vi "Equipment.vi"(8 "Error In":errorcluster, 11 "Equipment in":T1) -> (0 "Error Out":errorcluster, 3 "Equipment out":T1)   [LabVIEW 2018]
uses:
  Equipment.ctl
panel:
  in  "IMEI":string caption="String"
  in  "Serial Number":string caption="String"
  in  "Manufacturer":string caption="String"
  in  "Model":string caption="String"
  in  "Trademark":string caption="String"
  in  "Equipment":string caption="String"
  in  "Save":bool
  # "Equipment:"
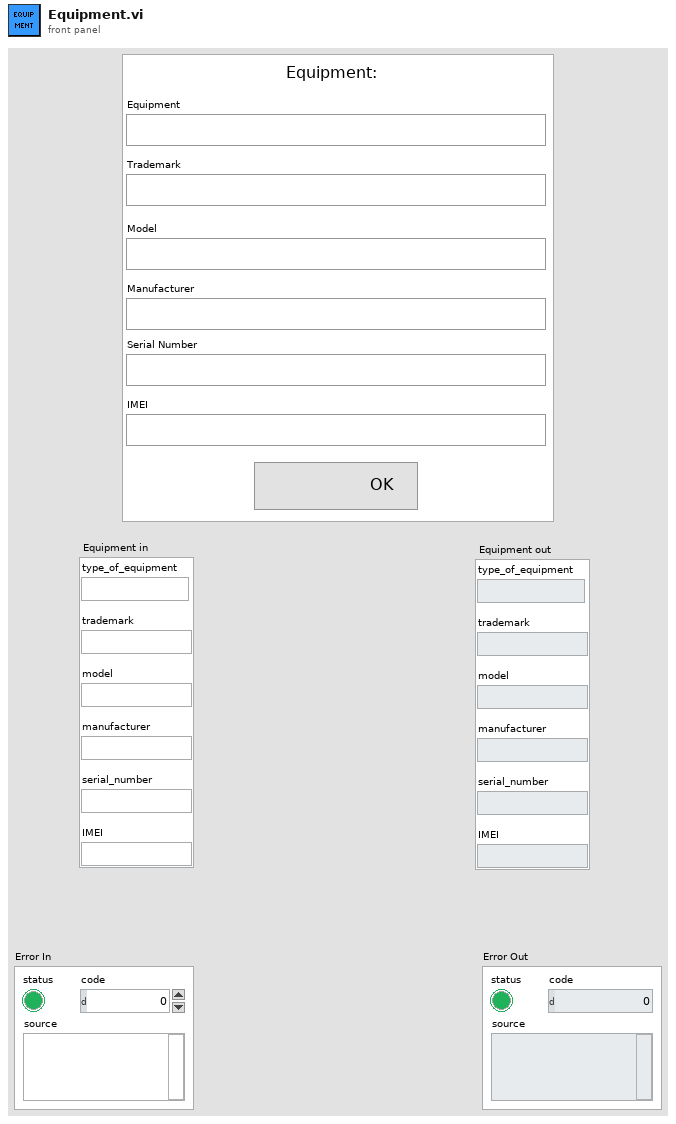
[diagram p1: front panel]
types:
  T1 = typedef "Equipment.ctl" = cluster{"type_of_equipment":string, "trademark":string, "model":string, "manufacturer":string, "serial_number":string, "IMEI":string}
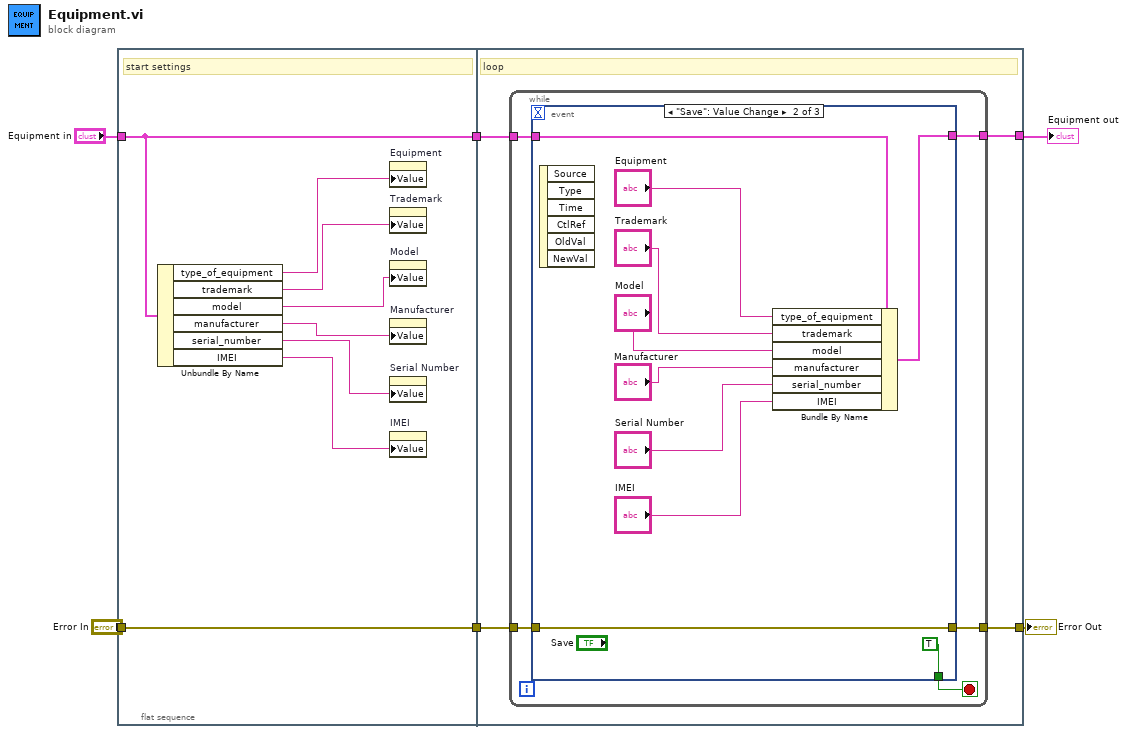
[diagram p0: block diagram]
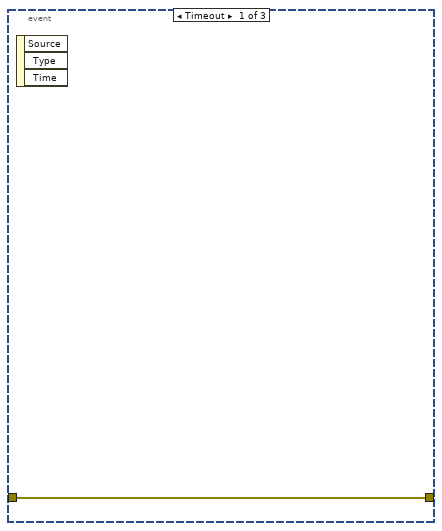
[diagram p2: hidden frame]
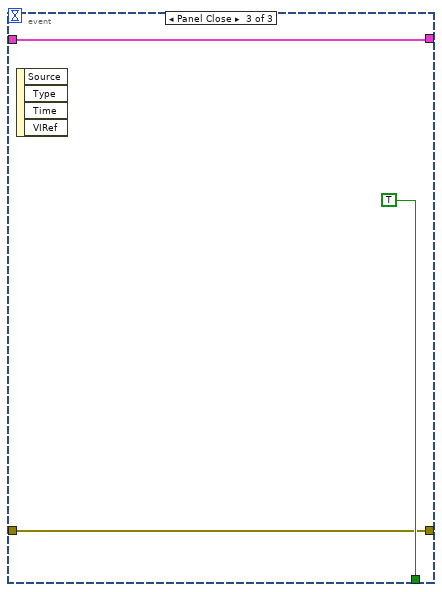
[diagram p3: hidden frame]
diagram:
  n1 = flat-sequence {
    tunnel: [w14] -> w6
    tunnel: "Equipment in" -> [w14]
    tunnel: [w13] -> w4
    tunnel: "Error In" -> [w13]
    tunnel: w6 -> [w18]
    tunnel: [w17] -> w1
    tunnel: w4 -> [w15]
    tunnel: [w16] -> w2
    frame #0 {
      # "start settings"
      n2 = Unbundle By Name(w14) -> ("type_of_equipment"=w12:string, "trademark"=w11:string, "model"=w10:string, "manufacturer"=w9:string, "serial_number"=w8:string, "IMEI"=w7:string)
      n3 = property on="Equipment" class="Str"("Value"=w12) -> ()  [unwired: 2 in, 2 out]
      n4 = property on="Trademark" class="Str"("Value"=w11) -> ()  [unwired: 2 in, 2 out]
      n5 = property on="Model" class="Str"("Value"=w10) -> ()  [unwired: 2 in, 2 out]
      n6 = property on="Manufacturer" class="Str"("Value"=w9) -> ()  [unwired: 2 in, 2 out]
      n7 = property on="Serial Number" class="Str"("Value"=w8) -> ()  [unwired: 2 in, 2 out]
      n8 = property on="IMEI" class="Str"("Value"=w7) -> ()  [unwired: 2 in, 2 out]
    }
    frame #1 {
      # "loop"
      n9 = while {
        tunnel: w18 -> [w22]
        tunnel: [w21] -> w17
        tunnel: [w20] -> w16
        tunnel: w15 -> [w19]
        stop <- w23 stop-if-true
        n10 = event shown="[1] \"Save\": Value Change" {
          selector: _ -> [_ _ _]
          dyn-events: _ -> [_ _ _]
          timeout: _ -> [_ _ _]
          tunnel: [_ TRUE TRUE] -> w23
          tunnel: w22 -> [_ w33 w36]
          tunnel: [_ w32 w36] -> w21
          tunnel: [w24 w31 w35] -> w20
          tunnel: w19 -> [w24 w31 w35]
          event Timeout {
            n11 = event-data() -> ()  [unwired: 1 in, 3 out]
          }
          event "Save": Value Change {
            n12 = event-data() -> ()  [unwired: 1 in, 6 out]
            n13 = Bundle By Name(cluster=w33, "type_of_equipment"="Equipment", "trademark"="Trademark", "model"="Model", "manufacturer"="Manufacturer", "serial_number"="Serial Number", "IMEI"="IMEI") -> (w32:T1)
          }
          event Panel Close {
            n14 = event-data() -> ()  [unwired: 1 in, 4 out]
          }
        }
      }
    }
  }
  "Error Out" <- w2
  "Equipment out" <- w1
